vi "Remove Duplicates from Color Array.vi"(11 "Array In":i32[][](array[numeric])) -> (3 "Array Out":i32[][](array[numeric]))   [LabVIEW 2021, in "lv_icon.lvlib"]
doc: "Removes duplicates from a color array. That usually happens when the Fill Algorithm visits the same pixel multiple times.s"
uses:
  lv_icon.lvlib
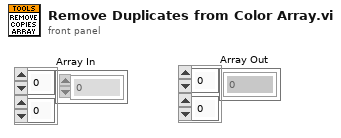
[diagram p1: front panel]
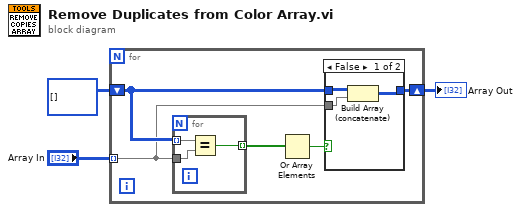
[diagram p0: block diagram]
diagram:
  n1 = for {
    tunnel: "Array In" -> [w4] mode=indexing
    shift-right: [w5] -> w3
    shift-left: i32[][] [] -> [w6]
    n2 = for {
      tunnel: w6 -> [w15] mode=indexing
      tunnel: w4 -> [w14]
      tunnel: [w13] -> w8 mode=indexing
      n3 = Equal?(x=w15, y=w14) -> (x = y?=w13:bool)
    }
    n4 = Or Array Elements(Boolean array=w8) -> (logical OR=w7:bool)
    n5 = case shown="False" w7 {
      tunnel: w6 -> [w11 w12]
      tunnel: [w10 w12] -> w5
      tunnel: w4 -> [w9 _]
      frame False {
        n6 = Build Array (concatenate)(w11, w9) -> (w10:i32[][])
      }
      frame True {
      }
    }
  }
  "Array Out" <- w3
